vi "demo.vi"() -> (0 "Error Out":errorcluster)   [LabVIEW 2024]
uses:
  Source/Instrument Manager/Instrument Manager.lvclass
  Source/Interfaces/IRunnable/IRunnable.lvclass
  Source/Interfaces/IRead Temperature/IRead Temperature.lvclass
  Source/Interfaces/IReadPressure/IRead Pressure.lvclass
  Source/Interfaces/IRead Dew Point/IRead Dew Point.lvclass
  Source/Interfaces/IRead Humidity/IRead Humidity.lvclass
  Source/Interfaces/IRead H2O Concentration/IRead H2O Concentration.lvclass
  Source/Interfaces/IVirtual Instrument/IVirtual Instrument.lvclass
  Alarming-Actor/Source/Alarming Actor/Alarming Actor/Alarming Actor.lvclass
  Alarming-Actor/Source/Alarming Actor UI/Alarming Actor UI.lvclass
  Alarming-Actor/Source/Alarming Actor/Alarming Actor/Alarming Level.ctl
panel:
  out "Identifier":string
  out "Alarming Level":T1
  out "Temperature":dbl format="%.2f °C"
  out "Time Stamp t":timestamp format="%<%x %.3X>T"
  in  "stop":bool
  out "Pressure":dbl format="%d mbar a"
  out "Time Stamp p":timestamp format="%<%x %.3X>T"
  out "Dew Point":dbl format="%.2f °C"
  out "Time Stamp d":timestamp format="%<%x %.3X>T"
  out "iteration":i32
  out "Absolute Humidity":dbl format="%.1f g/m³"
  out "Time Stamp h":timestamp format="%<%x %.3X>T"
  out "H2O Concentration":dbl format="%d Vol.-%"
  out "Time Stamp c":timestamp format="%<%x %.3X>T"
  out "Supply Chart":T2(graph)
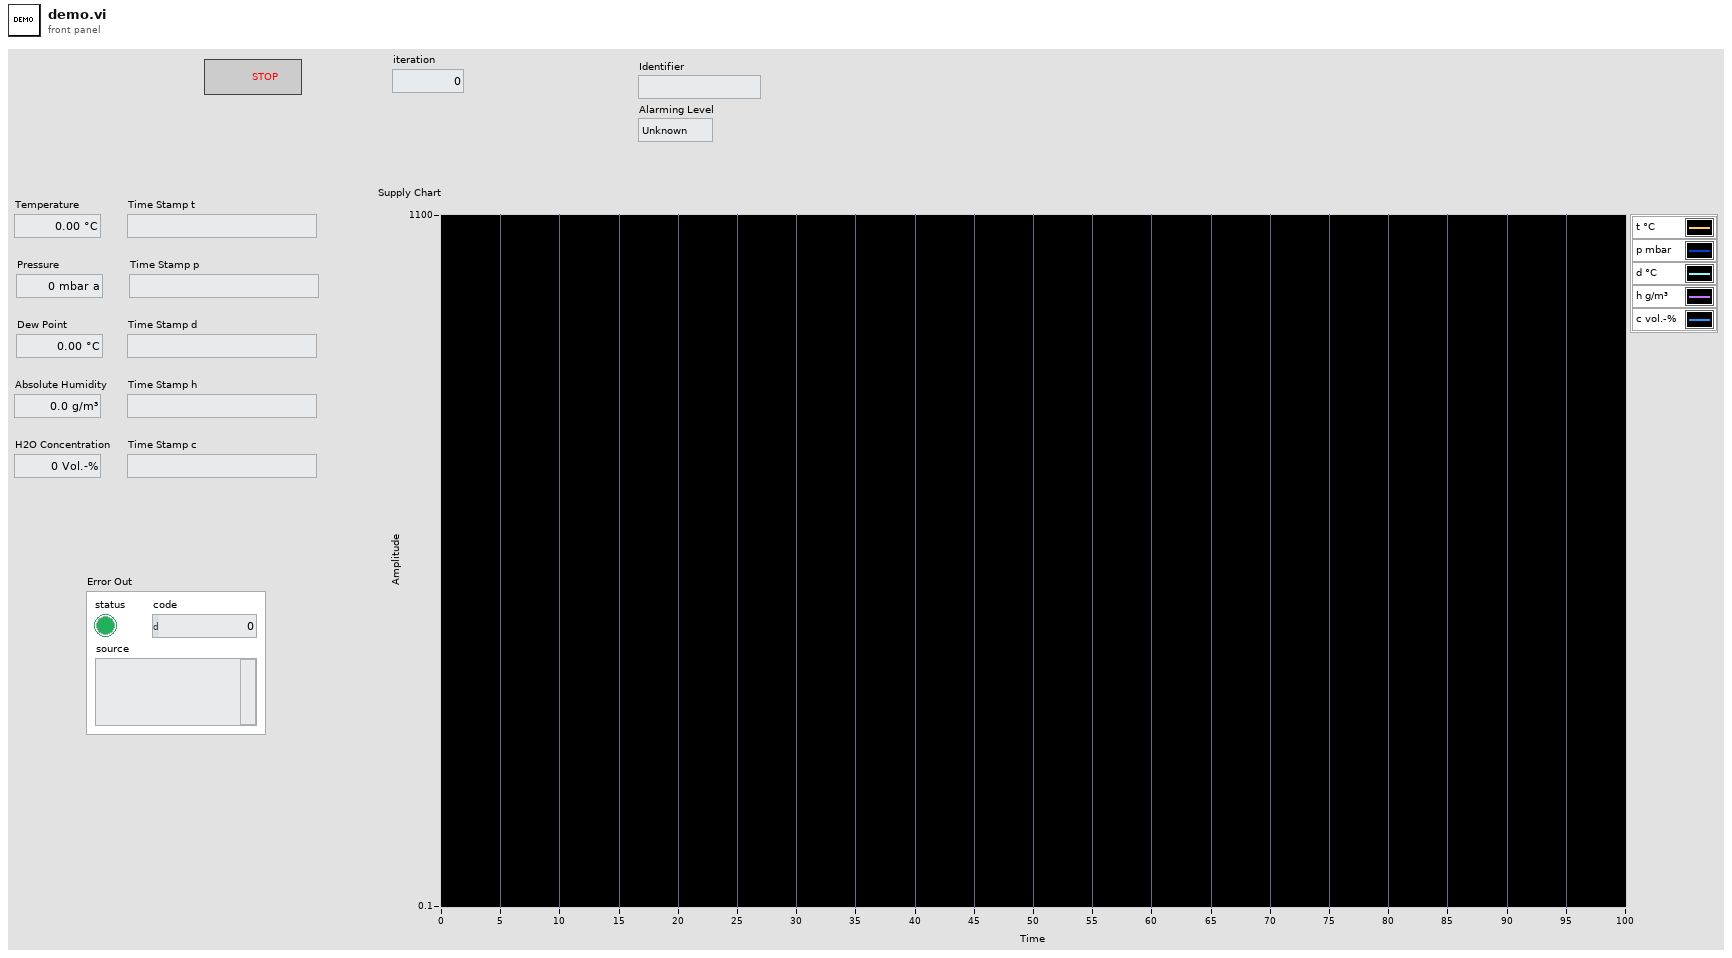
[diagram p1: front panel]
types:
  T1 = typedef "Alarming Actor.lvlib/Alarming Actor.lvclass/Alarming Level.ctl" = enum16{"Unknown", "OK", "Warning", "Critical"}
  T2 = cluster{"Temperature":dbl, "Pressure":dbl, "Dew Point":dbl, "Humidity":dbl, "H2O Concentration":dbl}
  T3 = cluster{"Identifier":string, "Alarming Level":T1}
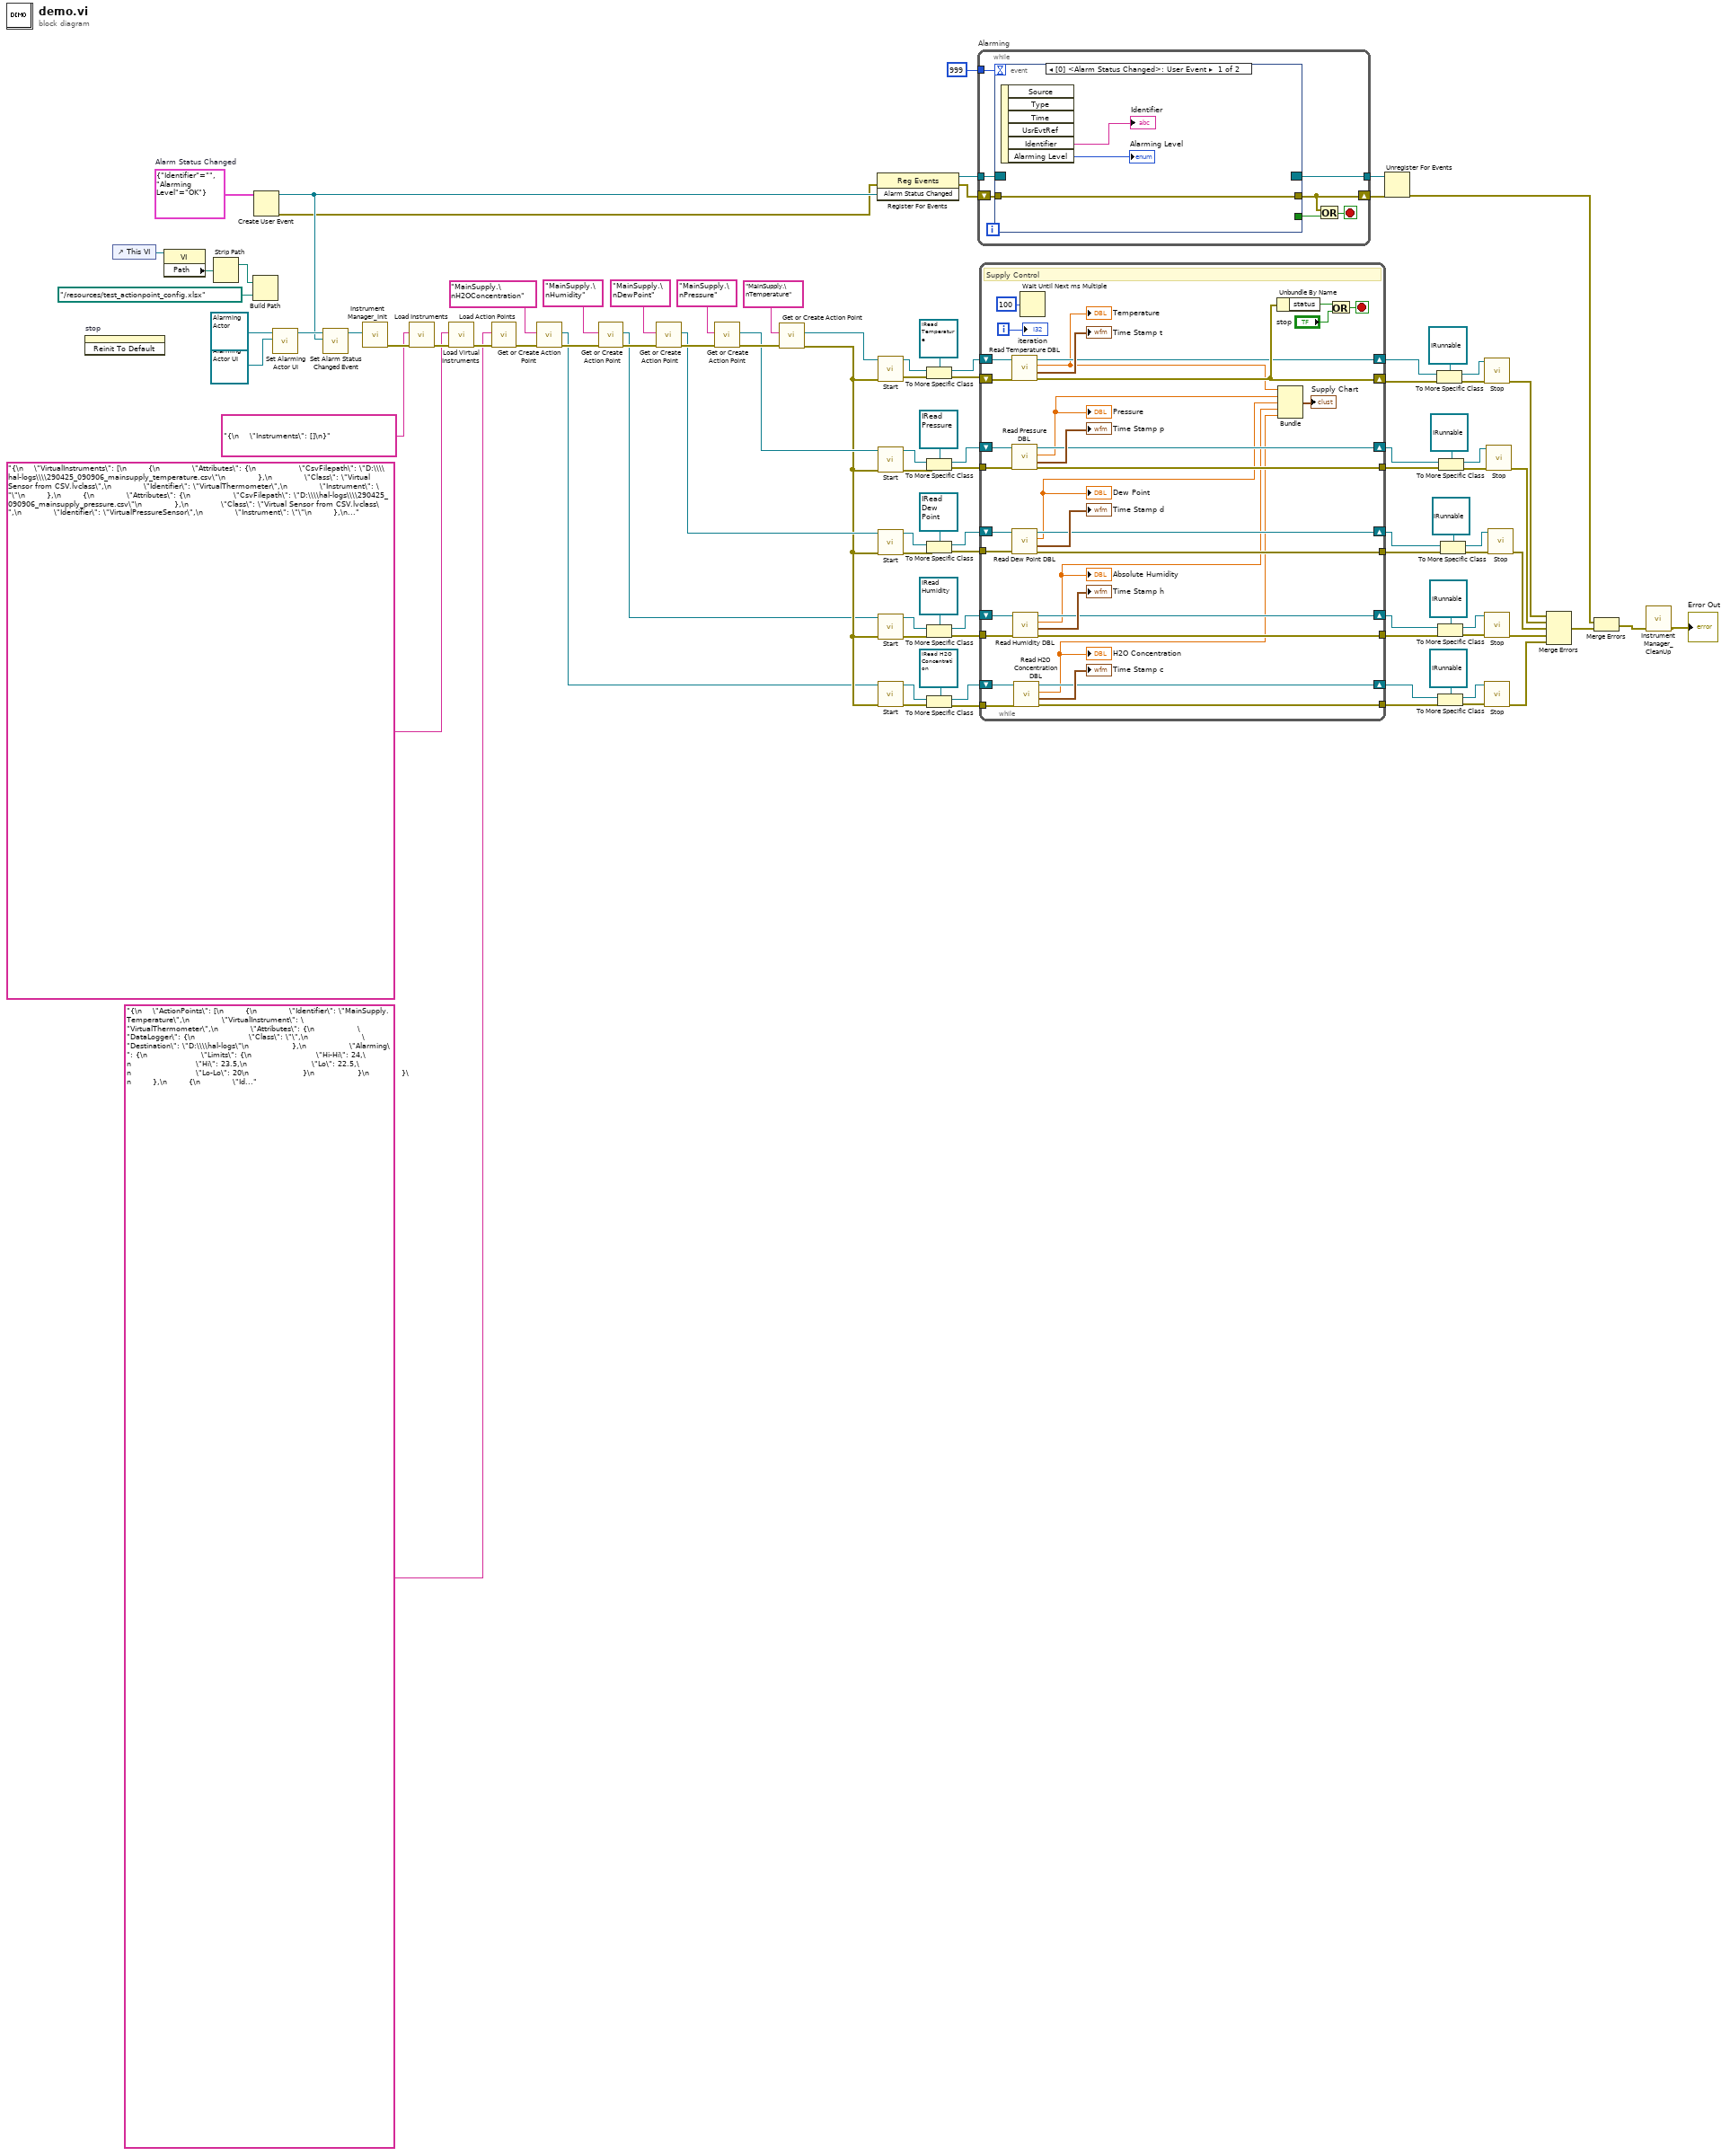
[diagram p0: block diagram]
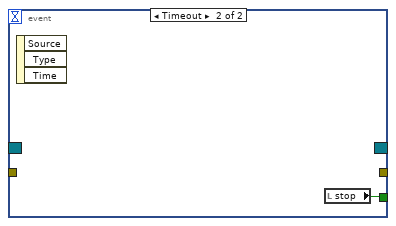
[diagram p2: hidden frame]
diagram:
  w12 = T3 {"Identifier"="", "Alarming Level"=enum."OK"}  # Alarm Status Changed
  n1 = invoke on="stop" class="Bool (strict)" method="Reinit To Default"() -> ()  [unwired: 3 in, 3 out]
  n2 = control-ref of="This VI"() -> (w52:refnum<vi>)
  n3 = property class="VI"(reference=w52) -> ("Path"=w51:path)  [unwired: 1 in, 2 out]
  n4 = Strip Path(path=w51) -> (stripped path=w19:path)  [unwired: 1 out]
  n5 = Build Path(base path=w19, name or relative path=path "../resources/test_actionpoint_config.xlsx") -> ()  [unwired: 1 out]
  n6 = Create User Event(user event datatype=w12) -> (user event=w9:refnum<user-event>, error out=w6:errorcluster)  [unwired: 1 in]
  n7 = call "Set Alarming Actor UI.vi"("UI Actor"=refnum<class "Alarming Actor UI.lvclass"> refnum ("Alarming Actor UI.lvlib:Alarming Actor UI.lvclass"), "Alarming Actor in"=refnum<class "Alarming Actor.lvclass"> refnum ("Alarming Actor.lvlib:Alarming Actor.lvclass")) -> ("Alarming Actor out"=w15:refnum<class "Alarming Actor.lvclass">)  [unwired: 9 in]
  n8 = call "Set Alarm Status Changed Event.vi"("Alarm Status Changed"=w9, "Alarming Actor in"=w15) -> ("Alarming Actor out"=w14:refnum<class "Alarming Actor.lvclass">)  [unwired: 9 in]
  n9 = call "Instrument Manager_Init.vi"("Alarming Actor"=w14) -> ("Error Out"=w96:errorcluster)  [unwired: 9 in, 1 out]
  n10 = call "Load Instruments.vi"("Error In"=w96, "Source"="{\n    \"Instruments\": []\n}") -> ("Error Out"=w94:errorcluster)  [unwired: 9 in]
  n11 = call "Load Virtual Instruments.vi"("Error In"=w94, "Source"="{\n    \"VirtualInstruments\": [\n        {\n            \"Attributes\": {\n                \"CsvFilepath\": \"D:\\\\hal-logs\\\\290425_090906_mainsupply_temperature.csv\"\n            },\n            \"Class\": \"Virtual Sensor from CSV.lvclass\",\n            \"Identifier\": \"VirtualThermometer\",\n            \"Instrument\": \"\"\n        },\n        {\n            \"Attributes\": {\n                \"CsvFilepath\": \"D:\\\\hal-logs\\\\290425_090906_mainsupply_pressure.csv\"\n            },\n            \"Class\": \"Virtual Sensor from CSV.lvclass\",\n            \"Identifier\": \"VirtualPressureSensor\",\n            \"Instrument\": \"\"\n        },\n        {\n            \"Attributes\": {\n                \"CsvFilepath\": \"D:\\\\hal-logs\\\\290425_090906_mainsupply_dewpoint.csv\"\n            },\n            \"Class\": \"Virtual Sensor from CSV.lvclass\",\n            \"Identifier\": \"VirtualDewPointSensor\",\n            \"Instrument\": \"\"\n        },\n        {\n            \"Attributes\": {\n                \"CsvFilepath\": \"D:\\\\hal-logs\\\\290425_090906_mainsupply_humidity.csv\"\n            },\n            \"Class\": \"Virtual Sensor from CSV.lvclass\",\n            \"Identifier\": \"VirtualHumiditySensor\",\n            \"Instrument\": \"\"\n        },\n        {\n            \"Attributes\": {\n                \"CsvFilepath\": \"D:\\\\hal-logs\\\\290425_090906_mainsupply_h2oconcentration.csv\"\n            },\n            \"Class\": \"Virtual Sensor from CSV.lvclass\",\n            \"Identifier\": \"VirtualH2OConcentrationSensor\",\n            \"Instrument\": \"\"\n        }\n    ]\n}") -> ("Error Out"=w67:errorcluster)  [unwired: 9 in]
  n12 = call "Load Action Points.vi"("Error In"=w67, "Source"="{\n    \"ActionPoints\": [\n        {\n            \"Identifier\": \"MainSupply.Temperature\",\n            \"VirtualInstrument\": \"VirtualThermometer\",\n            \"Attributes\": {\n                \"DataLogger\": {\n                    \"Class\": \"\",\n                    \"Destination\": \"D:\\\\hal-logs\"\n                },\n                \"Alarming\": {\n                    \"Limits\": {\n                        \"Hi-Hi\": 24,\n                        \"Hi\": 23.5,\n                        \"Lo\": 22.5,\n                        \"Lo-Lo\": 20\n                    }\n                }\n            }\n        },\n        {\n            \"Identifier\": \"MainSupply.Pressure\",\n            \"VirtualInstrument\": \"VirtualPressureSensor\",\n            \"Attributes\": {\n                \"DataLogger\": {\n                    \"Class\": \"\",\n                    \"Destination\": \"D:\\\\hal-logs\"\n                },\n                \"Alarming\": {\n                    \"Limits\": {\n                        \"Hi-Hi\": 1021,\n                        \"Hi\": 1019,\n                        \"Lo\": 0,\n                        \"Lo-Lo\": 0\n                    }\n                }\n            }\n        },\n        {\n            \"Identifier\": \"MainSupply.DewPoint\",\n            \"VirtualInstrument\": \"VirtualDewPointSensor\",\n            \"Attributes\": {\n                \"DataLogger\": {\n                    \"Class\": \"\",\n                    \"Destination\": \"D:\\\\hal-logs\"\n                },\n                \"Alarming\": {\n                    \"Limits\": {\n                        \"Hi-Hi\": 9,\n                        \"Hi\": 7.5,\n                        \"Lo\": 7,\n                        \"Lo-Lo\": 5\n                    }\n                }\n            }\n        },\n        {\n            \"Identifier\": \"MainSupply.Humidity\",\n            \"VirtualInstrument\": \"VirtualHumiditySensor\",\n            \"Attributes\": {\n                \"DataLogger\": {\n                    \"Class\": \"\",\n                    \"Destination\": \"D:\\\\hal-logs\"\n                },\n                \"Alarming\": {\n                    \"Limits\": {\n                        \"Hi-Hi\": 10,\n                        \"Hi\": 8,\n                        \"Lo\": 6,\n                        \"Lo-Lo\": 4\n                    }\n                }\n            }\n        },\n        {\n            \"Identifier\": \"MainSupply.H2OConcentration\",\n            \"VirtualInstrument\": \"VirtualH2OConcentrationSensor\",\n            \"Attributes\": {\n                \"DataLogger\": {\n                    \"Class\": \"\",\n                    \"Destination\": \"D:\\\\hal-logs\"\n                },\n                \"Alarming\": {\n                    \"Limits\": {\n                        \"Hi-Hi\": 3,\n                        \"Hi\": 2,\n                        \"Lo\": 0,\n                        \"Lo-Lo\": 0\n                    }\n                }\n            }\n        }\n    ]\n}") -> ("Error Out"=w21:errorcluster)  [unwired: 9 in]
  n13 = call "Get or Create Action Point.vi"("Error In"=w21, "Action Point Identifier"="MainSupply.\nH2OConcentration" ("Virtual Instrument Identifier")) -> ("Error Out"=w25:errorcluster, "IAction Point"=w22:refnum<class "IVirtual Instrument.lvclass">)  [unwired: 8 in]
  n14 = call "Get or Create Action Point.vi"("Error In"=w25, "Action Point Identifier"="MainSupply.\nHumidity" ("Virtual Instrument Identifier")) -> ("Error Out"=w34:errorcluster, "IAction Point"=w23:refnum<class "IVirtual Instrument.lvclass">)  [unwired: 8 in]
  n15 = call "Get or Create Action Point.vi"("Error In"=w34, "Action Point Identifier"="MainSupply.\nDewPoint" ("Instrument Identifier")) -> ("Error Out"=w66:errorcluster, "IAction Point"=w62:refnum<class "IVirtual Instrument.lvclass">)  [unwired: 8 in]
  n16 = call "Get or Create Action Point.vi"("Error In"=w66, "Action Point Identifier"="MainSupply.\nPressure" ("Virtual Instrument Identifier")) -> ("Error Out"=w93:errorcluster, "IAction Point"=w68:refnum<class "IVirtual Instrument.lvclass">)  [unwired: 8 in]
  n17 = call "Get or Create Action Point.vi"("Error In"=w93, "Action Point Identifier"="MainSupply.\nTemperature" ("Instrument Identifier")) -> ("Error Out"=w36:errorcluster, "IAction Point"=w53:refnum<class "IVirtual Instrument.lvclass">)  [unwired: 8 in]
  n18 = register-events(error in=w6, w9) -> (reference out=w10:refnum<event-registration>, error out=w7:errorcluster)  [unwired: 1 in]
  n19 = call-dynamic "Start.vi"("error in"=w36, "IRunnable in"=w53) -> ("error out"=w86:errorcluster, "IRunnable out"=w87:refnum<class "IVirtual Instrument.lvclass">)  [unwired: 8 in]
  n20 = call-dynamic "Start.vi"("error in"=w36, "IRunnable in"=w68) -> ("error out"=w83:errorcluster, "IRunnable out"=w82:refnum<class "IVirtual Instrument.lvclass">)  [unwired: 8 in]
  n21 = call-dynamic "Start.vi"("error in"=w36, "IRunnable in"=w62) -> ("error out"=w73:errorcluster, "IRunnable out"=w74:refnum<class "IVirtual Instrument.lvclass">)  [unwired: 8 in]
  n22 = call-dynamic "Start.vi"("error in"=w36, "IRunnable in"=w23) -> ("error out"=w49:errorcluster, "IRunnable out"=w48:refnum<class "IVirtual Instrument.lvclass">)  [unwired: 8 in]
  n23 = call-dynamic "Start.vi"("error in"=w36, "IRunnable in"=w22) -> ("error out"=w37:errorcluster, "IRunnable out"=w35:refnum<class "IVirtual Instrument.lvclass">)  [unwired: 8 in]
  n24 = To More Specific Class(target class=refnum<class "IRead Temperature.lvclass"> refnum ("IRead Temperature.lvclass"), reference=w87, error in=w86) -> (specific class reference=w84:refnum<class "IRead Temperature.lvclass">, error out=w85:errorcluster)
  n25 = To More Specific Class(target class=refnum<class "IRead Pressure.lvclass"> refnum ("IRead Pressure.lvclass"), reference=w82, error in=w83) -> (specific class reference=w70:refnum<class "IRead Pressure.lvclass">, error out=w69:errorcluster)
  n26 = To More Specific Class(target class=refnum<class "IRead Dew Point.lvclass"> refnum ("IRead Dew Point.lvclass"), reference=w74, error in=w73) -> (specific class reference=w71:refnum<class "IRead Dew Point.lvclass">, error out=w72:errorcluster)
  n27 = To More Specific Class(target class=refnum<class "IRead Humidity.lvclass"> refnum ("IRead Humidity.lvclass"), reference=w48, error in=w49) -> (specific class reference=w45:refnum<class "IRead Humidity.lvclass">, error out=w46:errorcluster)
  n28 = To More Specific Class(target class=refnum<class "IRead H2O Concentration.lvclass"> refnum ("IRead H2O Concentration.lvclass"), reference=w35, error in=w37) -> (specific class reference=w33:refnum<class "IRead H2O Concentration.lvclass">, error out=w38:errorcluster)
  n29 = while "Alarming" {
    shift-right: [w99] -> w8
    shift-left: w7 -> [w102]
    tunnel: w10 -> [w104]
    tunnel: [w103] -> w11
    tunnel: 999 -> [w98]
    stop <- w100 stop-if-true
    n30 = event shown="[0] <Alarm Status Changed>: User Event" {
      selector: w104 -> [_ _]
      dyn-events: [_ _] -> w103
      timeout: w98 -> [_ _]
      tunnel: w102 -> [w107 _]
      tunnel: [w107 _] -> w99
      tunnel: [_ w108] -> w101
      event User Event {
        n31 = event-data() -> ("Identifier"=→"Identifier":string, "Alarming Level"=→"Alarming Level":T1)  [unwired: 1 in, 4 out]
      }
      event Timeout {
        n32 = event-data() -> ()  [unwired: 1 in, 3 out]
        n33 = local read "stop"() -> (w108:bool)
      }
    }
    n34 = Or(x=w99, y=w101) -> (x .or. y?=w100:bool)
  }
  n35 = while {
    shift-right: [w138] -> w91
    shift-left: w84 -> [w136]
    shift-right: [w139] -> w97
    shift-left: w85 -> [w137]
    tunnel: w72 -> [w133]
    tunnel: w69 -> [w130]
    tunnel: [w129] -> w55
    tunnel: [w126] -> w58
    tunnel: w46 -> [w124]
    tunnel: [w122] -> w44
    tunnel: w38 -> [w119]
    tunnel: [w117] -> w28
    shift-right: [w128] -> w56
    shift-left: w70 -> [w131]
    shift-right: [w127] -> w57
    shift-left: w71 -> [w132]
    shift-right: [w120] -> w43
    shift-left: w45 -> [w123]
    shift-right: [w115] -> w20
    shift-left: w33 -> [w116]
    i -> [w125]
    stop <- w142 stop-if-true
    # "Supply Control"
    n36 = call-dynamic "Read Temperature DBL.vi"("error in"=w137, "IRead Temperature in"=w136) -> ("error out"=w139:errorcluster, "Time Stamp"=→"Time Stamp t":timestamp, "Temperature"=w114:dbl, "IRead Temperature out"=w138:refnum<class "IRead Temperature.lvclass">)  [unwired: 6 in]
    "Temperature" <- w114
    n37 = call-dynamic "Read Pressure DBL.vi"("error in"=w130, "IRead Pressure in"=w131) -> ("error out"=w129:errorcluster, "Time Stamp"=→"Time Stamp p":timestamp, "Pressure"=w113:dbl, "IRead Pressure out"=w128:refnum<class "IRead Pressure.lvclass">)  [unwired: 6 in]
    "Pressure" <- w113
    n38 = call-dynamic "Read Dew Point DBL.vi"("error in"=w133, "IRead Dew Point in"=w132) -> ("error out"=w126:errorcluster, "Time Stamp"=→"Time Stamp d":timestamp, "Dew Point"=w112:dbl, "IRead Dew Point out"=w127:refnum<class "IRead Dew Point.lvclass">)  [unwired: 6 in]
    "Dew Point" <- w112
    n39 = call-dynamic "Read Humidity DBL.vi"("error in"=w124, "IRead Absolute Humidity in"=w123) -> ("error out"=w122:errorcluster, "Time Stamp"=→"Time Stamp h":timestamp, "Humidity"=w111:dbl, "IRead Absolute Humidity out"=w120:refnum<class "IRead Humidity.lvclass">)  [unwired: 6 in]
    "Absolute Humidity" <- w111
    n40 = call-dynamic "Read H2O Concentration DBL.vi"("error in"=w119, "IRead Water Concentration in"=w116) -> ("error out"=w117:errorcluster, "Time Stamp"=→"Time Stamp c":timestamp, "H2O Concentration"=w110:dbl, "IRead Water Concentration out"=w115:refnum<class "IRead H2O Concentration.lvclass">)  [unwired: 6 in]
    "H2O Concentration" <- w110
    n41 = Wait Until Next ms Multiple(millisecond multiple=u32 100) -> ()  [unwired: 1 out]
    n42 = Unbundle By Name(w139) -> ("status"=w140:bool)
    n43 = Bundle("Temperature"=w114, "Pressure"=w113, "Dew Point"=w112, "Humidity"=w111, "H2O Concentration"=w110) -> (→"Supply Chart":T2)  [unwired: 1 in]
    n44 = Or(x=w140, y="stop") -> (x .or. y?=w142:bool)
    "iteration" <- w125
  }
  n45 = Unregister For Events(event registration refnum=w11, error in=w8) -> (error out=w1:errorcluster)
  n46 = To More Specific Class(target class=refnum<class "IRunnable.lvclass"> refnum ("IRunnable.lvclass"), reference=w91, error in=w97) -> (specific class reference=w89:refnum<class "IRunnable.lvclass">, error out=w92:errorcluster)
  n47 = To More Specific Class(target class=refnum<class "IRunnable.lvclass"> refnum ("IRunnable.lvclass"), reference=w43, error in=w44) -> (specific class reference=w40:refnum<class "IRunnable.lvclass">, error out=w42:errorcluster)
  n48 = To More Specific Class(target class=refnum<class "IRunnable.lvclass"> refnum ("IRunnable.lvclass"), reference=w20, error in=w28) -> (specific class reference=w30:refnum<class "IRunnable.lvclass">, error out=w29:errorcluster)
  n49 = To More Specific Class(target class=refnum<class "IRunnable.lvclass"> refnum ("IRunnable.lvclass"), reference=w56, error in=w55) -> (specific class reference=w80:refnum<class "IRunnable.lvclass">, error out=w78:errorcluster)
  n50 = To More Specific Class(target class=refnum<class "IRunnable.lvclass"> refnum ("IRunnable.lvclass"), reference=w57, error in=w58) -> (specific class reference=w59:refnum<class "IRunnable.lvclass">, error out=w61:errorcluster)
  n51 = call-dynamic "Stop.vi"("error in"=w92, "IRunnable in"=w89) -> ("error out"=w95:errorcluster)  [unwired: 8 in, 1 out]
  n52 = call-dynamic "Stop.vi"("error in"=w42, "IRunnable in"=w40) -> ("error out"=w41:errorcluster)  [unwired: 8 in, 1 out]
  n53 = call-dynamic "Stop.vi"("error in"=w29, "IRunnable in"=w30) -> ("error out"=w27:errorcluster)  [unwired: 8 in, 1 out]
  n54 = call-dynamic "Stop.vi"("error in"=w78, "IRunnable in"=w80) -> ("error out"=w76:errorcluster)  [unwired: 8 in, 1 out]
  n55 = call-dynamic "Stop.vi"("error in"=w61, "IRunnable in"=w59) -> ("error out"=w54:errorcluster)  [unwired: 8 in, 1 out]
  n56 = Merge Errors(w95, w76, w54, w41, w27) -> (w77:errorcluster)
  n57 = Merge Errors(w1, w77) -> (w2:errorcluster)
  n58 = call "Instrument Manager_CleanUp.vi"("Error In"=w2) -> ("Error Out"=→"Error Out":errorcluster)  [unwired: 10 in]
